vi "CopySRNumToClipboard.vi"(7 "SR Cloumn Header":string, 8 "Error In":errorcluster, 9 "Coordinates":T1, 11 "Table Reference":refnum<vi>) -> (0 "Error Out":errorcluster)   [LabVIEW 2017, in "Client.lvlib"]
uses:
  Client.lvlib
  <vilib>/Utility/miscctls.llb/LVPoint32TypeDef.ctl
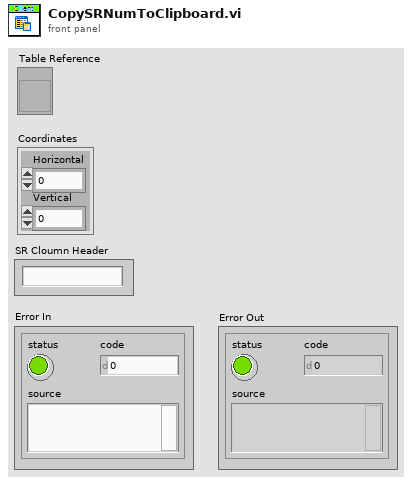
[diagram p1: front panel]
types:
  T1 = typedef "LVPoint32TypeDef.ctl" = cluster{"Horizontal":i32, "Vertical":i32}
  T2 = typedef "LVRowAndColumnTypeDef.ctl" = cluster{"Row":i32, "Column":i32}
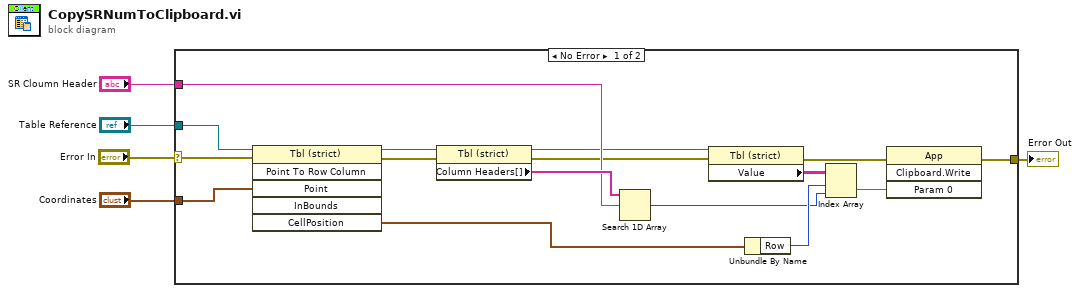
[diagram p0: block diagram]
diagram:
  n1 = case shown="No Error" "Error In" {
    selector: "Error In" -> [w7 w22]
    tunnel: "Coordinates" -> [w20 _]
    tunnel: "Table Reference" -> [w19 _]
    tunnel: "SR Cloumn Header" -> [w16 _]
    tunnel: [w6 w22] -> w1
    frame No Error {
      n2 = invoke class="Tbl (strict)" method="Point To Row Column"(reference=w19, error in=w7, "Point"=w20) -> (reference out=w18:refnum<vi>, error out=w14:errorcluster, "CellPosition"=w21:T2)  [unwired: 3 in, 3 out]
      n3 = property class="Tbl (strict)"(reference=w18, error in=w14) -> (reference out=w15:refnum<vi>, error out=w13:errorcluster, "Column Headers[]"=w17:string[])
      n4 = Search 1D Array(1D array=w17, element=w16) -> (index of element=w10:i32)  [unwired: 1 in]
      n5 = property class="Tbl (strict)"(reference=w15, error in=w13) -> (error out=w8:errorcluster, "Value"=w12:string[][])  [unwired: 1 out]
      n6 = Unbundle By Name(w21) -> ("Row"=w11:i32)
      n7 = Index Array(array=w12, index (row)=w11, index (col)=w10) -> (element=w9:string)
      n8 = invoke class="App" method="Clipboard.Write"(error in=w8, "Param 0"=w9) -> (error out=w6:errorcluster)  [unwired: 2 in, 3 out]
    }
    frame Error {
    }
  }
  "Error Out" <- w1
